vi "Main.vi"(8 "error":errorcluster) -> (0 "Error out":errorcluster)   [LabVIEW 2018, in "GUI.lvclass"]
uses:
  GUI.lvclass
  Public Controls/GlobalConfig.ctl
  Public Controls/S1Config.ctl
  Public Controls/S2Config.ctl
  Public Controls/TestInfo.ctl
  GUI.lvclass/GUI.ctl
  <vilib>/DAQmx/write.llb/DAQmx Write (Digital Bool 1Line 1Point).vi
  <vilib>/DAQmx/miscellaneous.llb/DAQmx Fill In Error Info.vi
  S1/S1.lvclass
  S2/S2.lvclass
  IO/IO.lvclass
  S3/S3.lvclass
  S4/S4.lvclass
  S5/S5.lvclass
  S6/S6.lvclass
  Serial/Serial.lvclass
panel:
  in  "Tab Control":T1(tab)
  out "S2 Valves":bool[](array[boolean])
  out "S1 Valves":bool[](array[boolean])
  out "EC_PTEST_DELTA_MAX":dbl format="%.2f psig"
  in  "S2AckAlarm":bool
  in  "S1AckAlarm":bool
  out "PRESSURE PT1":dbl(knob) scale=0.0..400.0
  out "PRESSURE PT1":dbl(knob) scale=0.0..400.0 scale format="%_3g"
  in  "ABORT1":bool
  out "ELAPSED TIME 2":dbl caption="REMAINING STATE TIME" format="%<%H:%M:%S>t"
  out "IsLidLocked 2":bool caption="IsLidLocked"
  in  "SN 2":string caption="SN"
  in  "S2Start":bool
  out "IsLidLocked":bool
  in  "S1Start":bool
  in  "SN":string
  in  "ABORT 2":bool
  out "ELAPSED TIME 1":dbl caption="REMAINING STATE TIME" format="%<%H:%M:%S>t"
  out "TEST STOPPED AT:":string
  out "S1 TEST STARTED AT:":string caption="TEST STARTED AT:"
  out "2 TEST STOPPED AT:":string caption="TEST STOPPED AT:"
  out "2 TEST STARTED AT:":string caption="TEST STARTED AT:"
  out "PRESSURE PT231":dbl(knob) scale=0.0..400.0
  out "PRESSURE PT221":dbl(knob) scale=0.0..400.0
  out "TEST RESULT 2":string caption="TEST RESULT"
  out "TEST STATE":string
  out "Pressure vs Time Plot 2":waveform(dbl)[](graph)
  out "TEST STATUS 2":string caption="TEST STATUS"
  in  "Select Test Type 2":string(combo) caption="Test Type"
  out "PRESSURE PT131":dbl(knob) scale=0.0..0.5 scale format="%_3g"
  out "PRESSURE PT121":dbl(knob) scale=0.0..400.0 scale format="%#.3g"
  out "PRESSURE PT111":dbl(knob) scale=0.0..400.0 scale format="%#.3g"
  out "TEST RESULT 1":string caption="TEST RESULT"
  out "CURRENT TEST STATE 1":string caption="TEST STATE"
  out "Pressure vs Time Plot 1":waveform(dbl)[](graph)
  out "TEST STATUS 1":string caption="TEST STATUS"
  in  "Test Type 1":string(combo) caption="Test Type"
  in  "LidLock-Extend(SV615)":bool
  in  "Z2 Vent(SV621)":bool
  in  "LidLock-Retract(SV614)":bool
  in  "Z3 Vent(SV633)":bool
  in  "Hi Pressure N2(SV632)":bool
  in  "Lo Pressure N2(SV631)":bool
  out "CPS612":bool
  out "CPS611":bool
  in  "LidLock-Extend(SV515)":bool
  in  "Z2 Vent(SV521)":bool
  in  "LidLock-Retract(SV514)":bool
  in  "Z3 Vent(SV533)":bool
  in  "Hi Pressure N2(SV532)":bool
  in  "Lo Pressure N2(SV531)":bool
  out "CPS512":bool
  out "CPS511":bool
  in  "LidLock-Extend(SV415)":bool
  in  "Z2 Vent(SV421)":bool
  in  "LidLock-Retract(SV414)":bool
  in  "Z3 Vent(SV433)":bool
  in  "Hi Pressure N2(SV432)":bool
  in  "Lo Pressure N2(SV431)":bool
  out "CPS412":bool
  out "CPS411":bool
  in  "LidLock-Extend(SV315)":bool
  in  "Z2 Vent(SV321)":bool
  in  "LidLock-Retract(SV314)":bool
  in  "Z3 Vent(SV333)":bool
  in  "Hi Pressure N2(SV332)":bool
  in  "Lo Pressure N2(SV331)":bool
  out "CPS312":bool
  out "CPS311":bool
  in  "LidLock-Extend(SV215)":bool
  in  "Z2 Vent(SV221)":bool
  in  "LidLock-Retract(SV214)":bool
  in  "Z3 Vent(SV233)":bool
  in  "LidLock-Retract(SV114)":bool
  in  "LidLock-Extend(SV115)":bool
  in  "Hi Pressure N2(SV232)":bool
  in  "Lo Pressure N2(SV231)":bool
  in  "Z3 Vent(SV131)":bool
  in  "Lo Pressure N2(SV111)":bool
  out "CPS212":bool
  out "CPS211":bool
  out "CPS112":bool
  out "CPS111":bool
  in  "Z1 Vent(SV113)":bool
  in  "Hi Pressure N2(SV112)":bool
  in  "Z2 Vent(SV121)":bool
  in  "Global":T2={"Report Folder Path"=path "", "PT1_MIN"=0.0, "PT1_MAX"=0.0, "VENT_PMAX"=0.0, "LOP_TARGET"=0.0, "LOP_RAMP"=0.0, "LOP_LEAK_MAX"=0.0, "HIP_TARGET"=0.0, "HIP_RAMP"=0.0, "HIP_MIN"=0.0, "HIP_MAX"=0.0, "BLEED_TIME"=0.0, "LOP_MAX"=0.0, "LOP_MIN"=0.0, "PT131Com"="COM5", "PT231Com"="COM6", "PT331Com"="COM7", "PT431Com"="COM8", "PT531Com"="COM9", "PT631Com"="COM10"} {"LOP_MIN" format="%#_g PSI"; "LOP_MAX" format="%#_g PSI"; "BLEED_TIME" format="%#_g Sec"; "HIP_MAX" format="%#_g PSI"; "HIP_MIN" format="%#_g PSI"; "HIP_RAMP" format="%#_g Sec"; "HIP_TARGET" format="%#_g PSI"; "LOP_LEAK_MAX" format="%#_g PSI"; "LOP_RAMP" format="%#_g Sec"; "LOP_TARGET" format="%#_g PSI"; "VENT_PMAX" format="%#_g PSI"; "PT1_MAX" format="%#_g PSI"; "PT1_MIN" format="%#_g PSI"}
  in  "S1Config":T3 {"TJHIP_STABLE_CLOSE" format="%#_g sec"; "TJHIP_STABLE_WAIT" format="%#_g sec"; "TJ_PTEST_MAX" format="%#_g in H20"; "TJHIP_TIMER" format="%#_g sec"; "TJLOP_TIMER" format="%#_g sec"; "MSHIP_TIMER" format="%#_g sec"; "S1Z3_LOP_LEAK_MAX" format="%#_g in H20"; "MSLOP_TIMER" format="%#_g sec"; "S1Z3_VENT_PMAX" format="%#_g in H20"}
  in  "Station 6":T4 {"EC_PTEST_DELTA_BASELINE" format="%#_g psi"; "EC_PTEST_SCALE_FACTOR" min=0.0 max=1.0 step=0.01; "ECZ3_POFF_STABLE" format="%#_g sec"; "EC_PSTABLE_WAIT" format="%#_g sec"; "EC_PTEST_TIMER" format="%#_g sec"; "ECLOP_TIMER" format="%#_g sec"}
  in  "Station 5":T4 {"EC_PTEST_DELTA_BASELINE" format="%#_g psi"; "EC_PTEST_SCALE_FACTOR" min=0.0 max=1.0 step=0.01; "ECZ3_POFF_STABLE" format="%#_g sec"; "EC_PSTABLE_WAIT" format="%#_g sec"; "EC_PTEST_TIMER" format="%#_g sec"; "ECLOP_TIMER" format="%#_g sec"}
  in  "Station 4":T4 {"EC_PTEST_DELTA_BASELINE" format="%#_g psi"; "EC_PTEST_SCALE_FACTOR" min=0.0 max=1.0 step=0.01; "ECZ3_POFF_STABLE" format="%#_g sec"; "EC_PSTABLE_WAIT" format="%#_g sec"; "EC_PTEST_TIMER" format="%#_g sec"; "ECLOP_TIMER" format="%#_g sec"}
  in  "Station 3":T4 {"EC_PTEST_DELTA_BASELINE" format="%#_g psi"; "EC_PTEST_SCALE_FACTOR" min=0.0 max=1.0 step=0.01; "ECZ3_POFF_STABLE" format="%#_g sec"; "EC_PSTABLE_WAIT" format="%#_g sec"; "EC_PTEST_TIMER" format="%#_g sec"; "ECLOP_TIMER" format="%#_g sec"}
  in  "Station 2":T4 {"EC_PTEST_DELTA_BASELINE" format="%#_g psi"; "EC_PTEST_SCALE_FACTOR" min=0.0 max=1.0 step=0.01; "ECZ3_POFF_STABLE" format="%#_g sec"; "EC_PSTABLE_WAIT" format="%#_g sec"; "EC_PTEST_TIMER" format="%#_g sec"; "ECLOP_TIMER" format="%#_g sec"}
  # "Version 2.0.0"
  # "This template is for the Simple State Machine design pattern.\n\nSee the block diagram for more information on how to use this template."
  # "STATION #1"
  # "STATION #2"
  # "LoP"
  # "HiP"
  # "Z1"
  # "Z2"
  # "Z3"
  # "Lid Ext"
  # "LoP"
  # "HiP"
  # "Z3"
  # "Z2"
  # "Lid Ext"
  # "STATION 1"
  # "STATION 2"
  # "STATION 4"
  # "STATION 5"
  # "STATION 6"
  # "STATION 3"
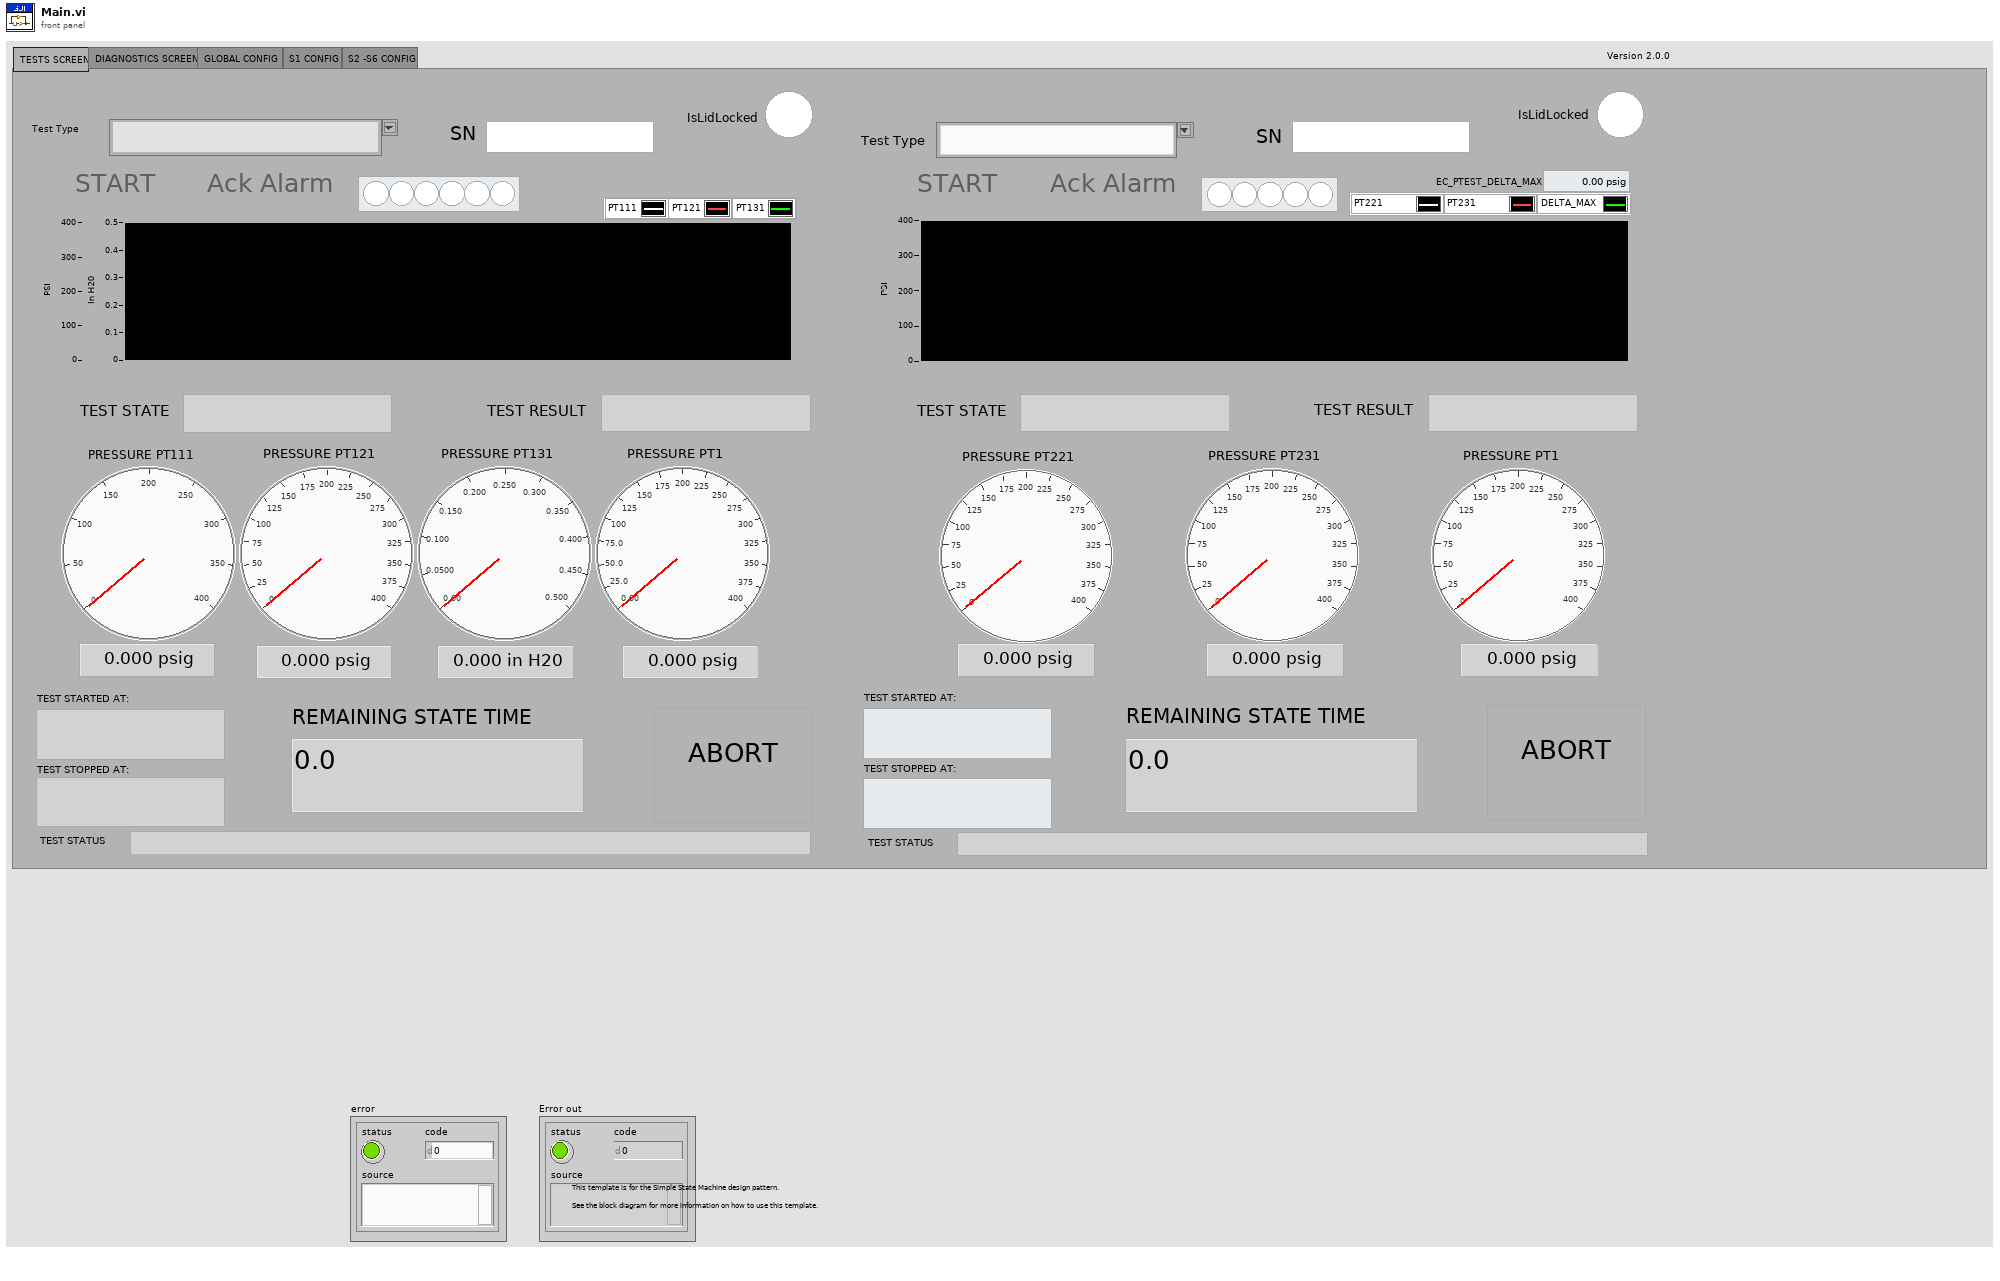
[diagram p1: front panel]
types:
  T1 = enum32{"TESTS SCREEN", "DIAGNOSTICS SCREEN", "GLOBAL CONFIG", "S1 CONFIG", "S2 -S6 CONFIG"}
  T2 = typedef "GUI.lvclass/GlobalConfig.ctl" = cluster{"Report Folder Path":path, "PT1_MIN":dbl, "PT1_MAX":dbl, "VENT_PMAX":dbl, "LOP_TARGET":dbl, "LOP_RAMP":dbl, "LOP_LEAK_MAX":dbl, "HIP_TARGET":dbl, "HIP_RAMP":dbl, "HIP_MIN":dbl, "HIP_MAX":dbl, "BLEED_TIME":dbl, "LOP_MAX":dbl, "LOP_MIN":dbl, "PT131Com":refnum<visa-resource-name>, "PT231Com":refnum<visa-resource-name>, "PT331Com":refnum<visa-resource-name>, "PT431Com":refnum<visa-resource-name>, "PT531Com":refnum<visa-resource-name>, "PT631Com":refnum<visa-resource-name>}
  T3 = typedef "GUI.lvclass/S1Config.ctl" = cluster{"S1Z3_VENT_PMAX":dbl, "MSLOP_TIMER":dbl, "S1Z3_LOP_LEAK_MAX":dbl, "MSHIP_TIMER":dbl, "TJLOP_TIMER":dbl, "TJHIP_TIMER":dbl, "TJ_PTEST_MAX":dbl, "TJHIP_STABLE_WAIT":dbl, "TJHIP_STABLE_CLOSE":dbl}
  T4 = typedef "GUI.lvclass/S2Config.ctl" = cluster{"ECLOP_TIMER":dbl, "EC_PTEST_TIMER":dbl, "EC_PSTABLE_WAIT":dbl, "ECZ3_POFF_STABLE":dbl, "EC_PTEST_SCALE_FACTOR":dbl, "EC_PTEST_DELTA_BASELINE":dbl}
  T5 = enum8{"Enabled", "Disabled", "Disabled and Grayed Out"}
  T6 = typedef "GUI.lvclass/TestInfo.ctl" = cluster{"TestType":string, "SN":string}
  T7 = typedef "GUI.lvclass/State.ctl" = enum16{"Initialize", "LoadConfig", "SaveConfig", "S1Alarm", "S2Alarm", "S1EndOfTest", "S2EndOfTest", "Monitor", "Error", "Exit"}
  T8 = cluster{"Global":T2, "S1Config":T3, "Station 2 ":T4, "Station 3":T4, "Station 4":T4, "Station 5":T4, "Station 6":T4}
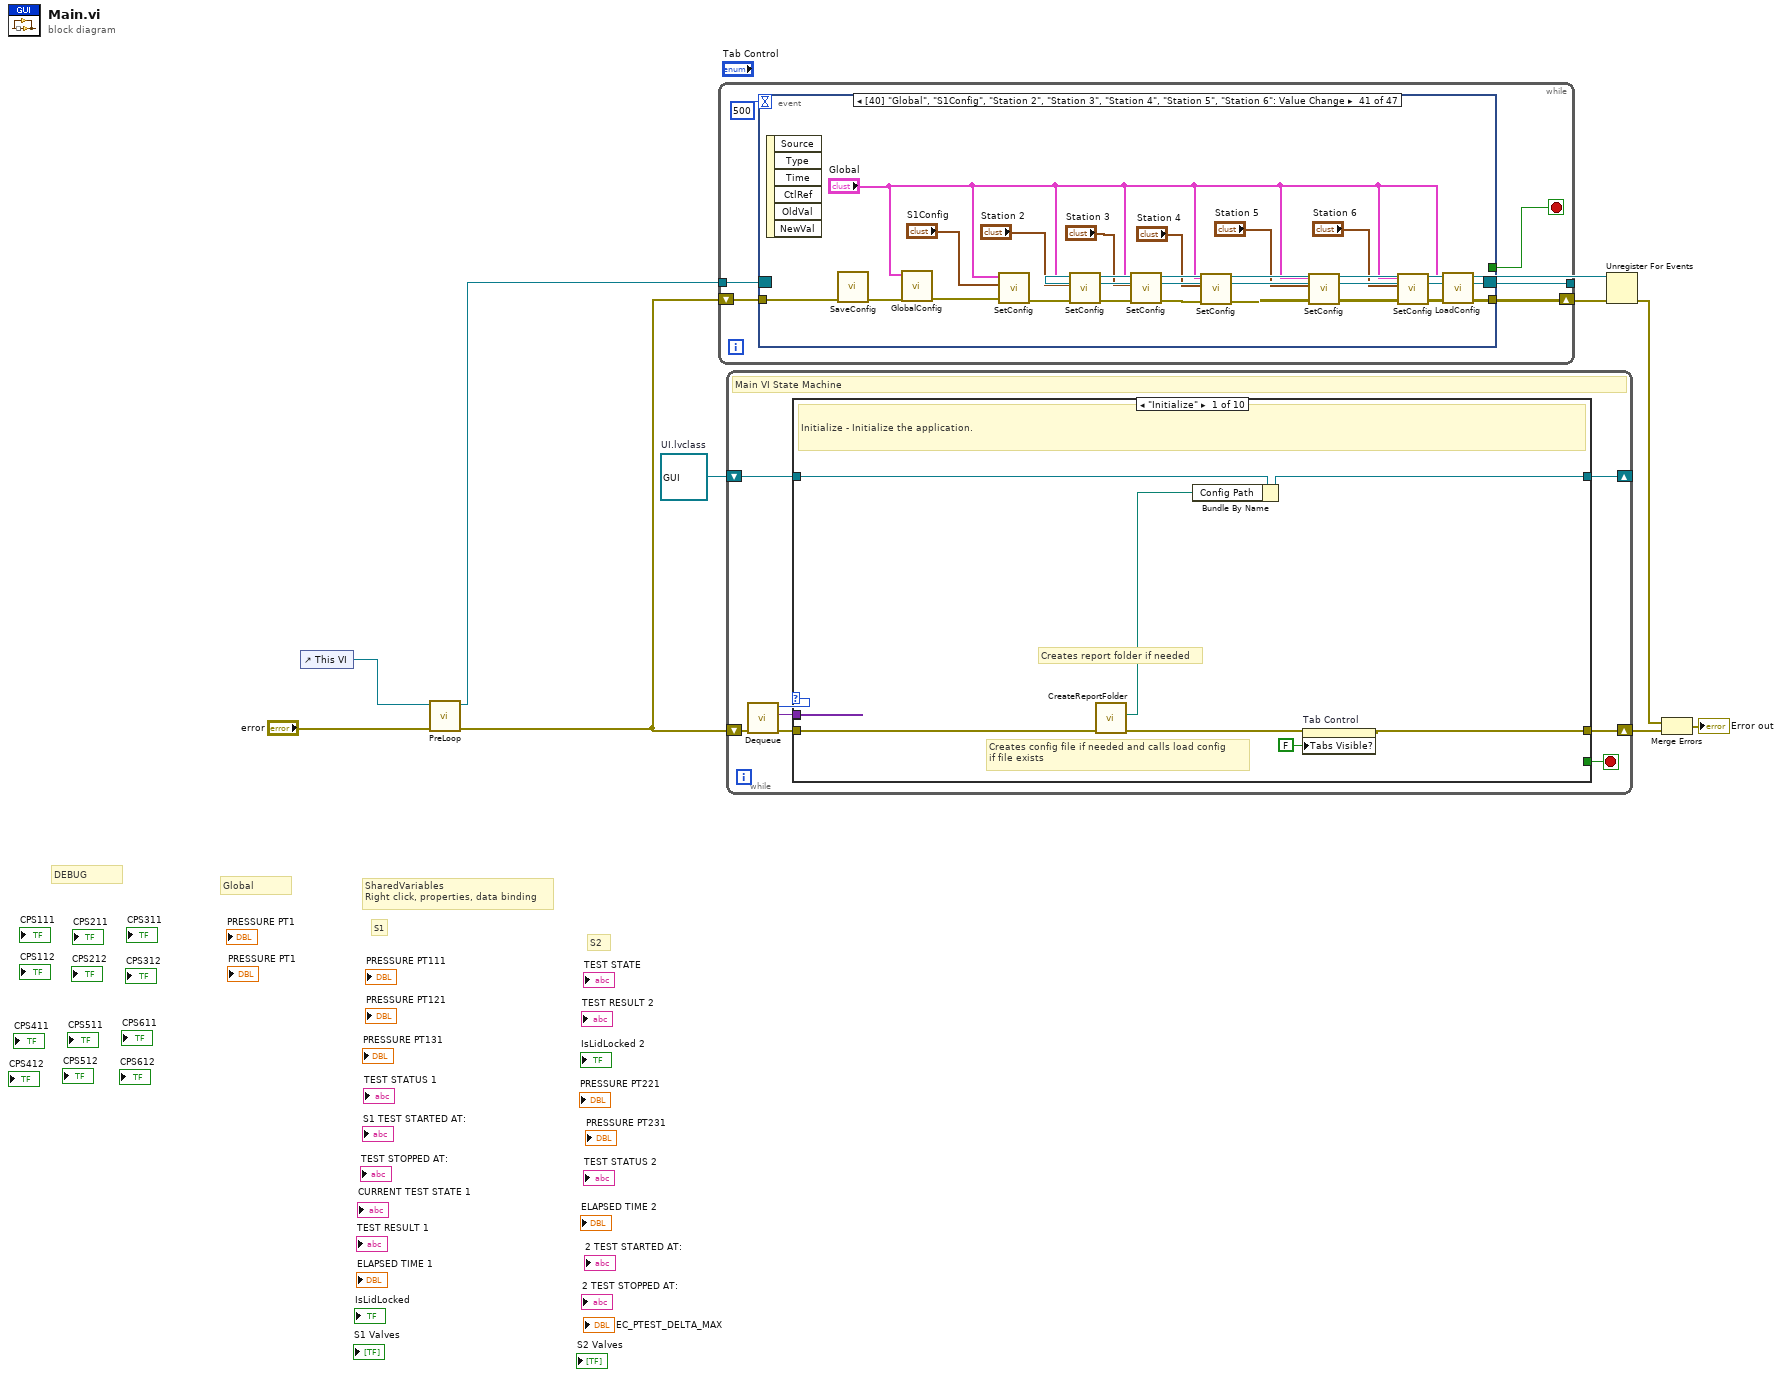
[diagram p0: block diagram]
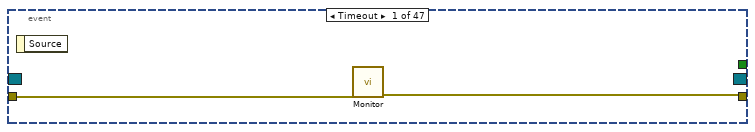
[diagram p2: hidden frame]
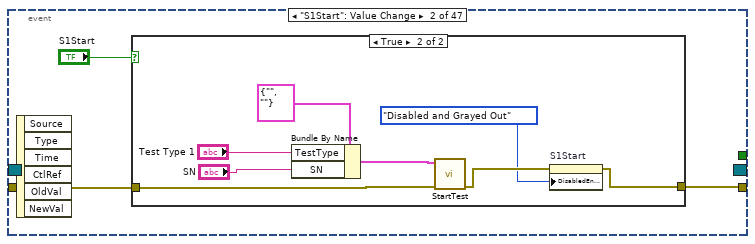
[diagram p3: hidden frame]
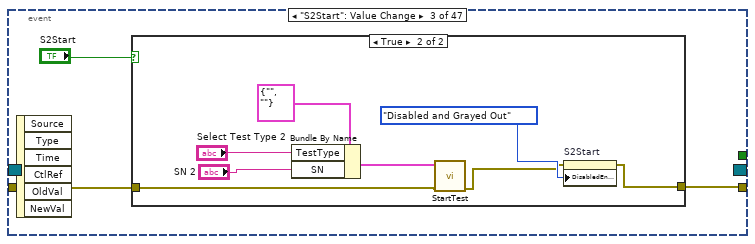
[diagram p5: hidden frame]
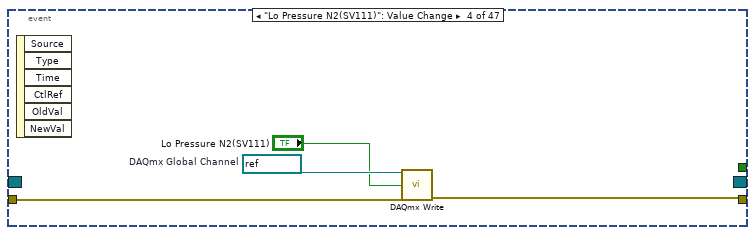
[diagram p7: hidden frame]
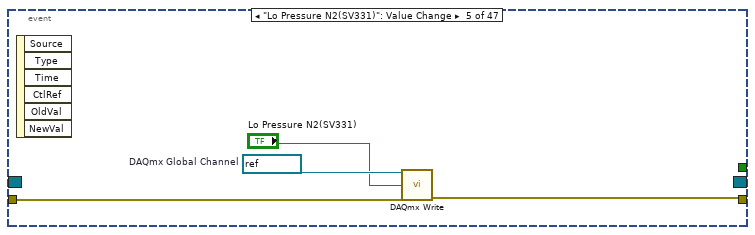
[diagram p8: hidden frame]
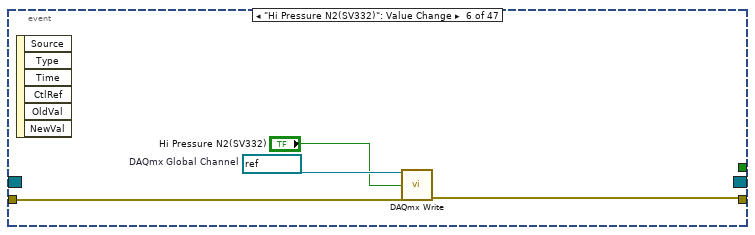
[diagram p9: hidden frame]
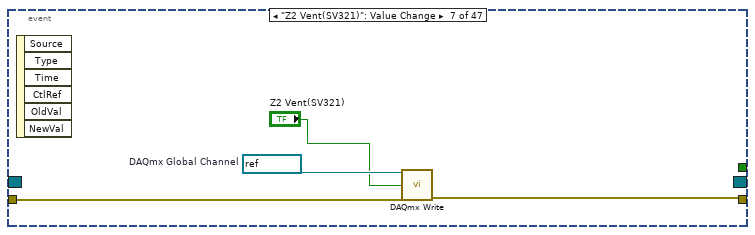
[diagram p10: hidden frame]
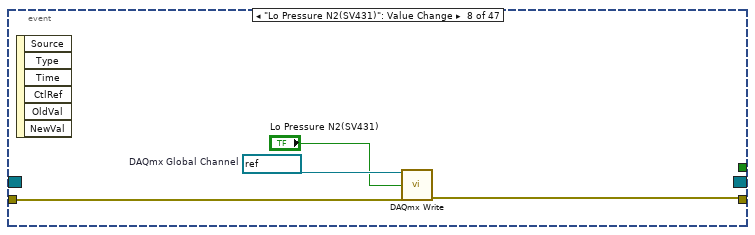
[diagram p11: hidden frame]
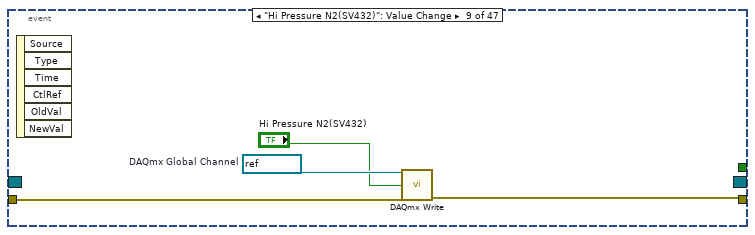
[diagram p12: hidden frame]
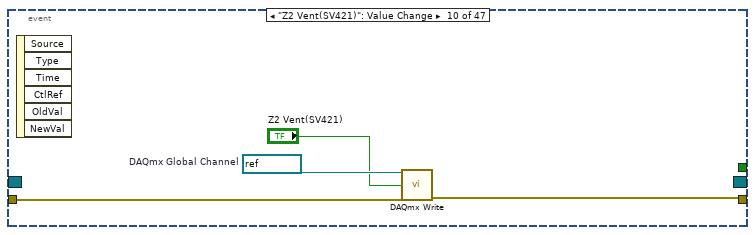
[diagram p13: hidden frame]
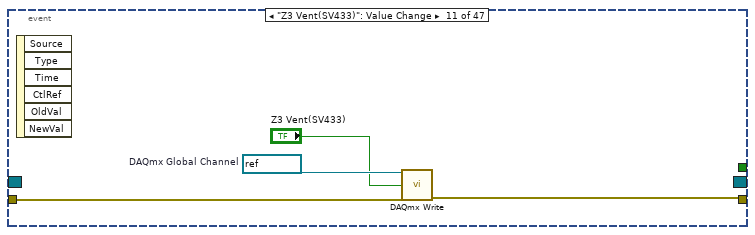
[diagram p14: hidden frame]
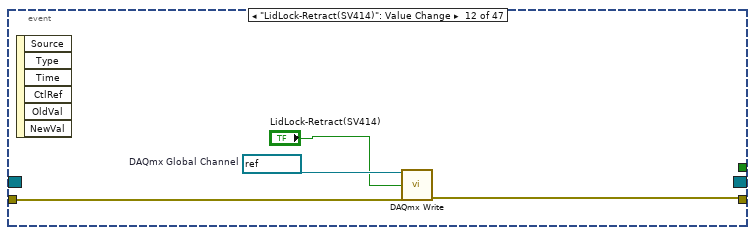
[diagram p15: hidden frame]
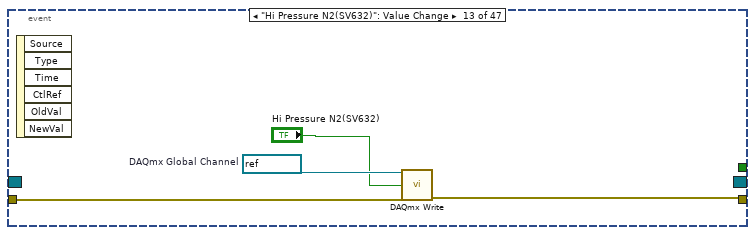
[diagram p16: hidden frame]
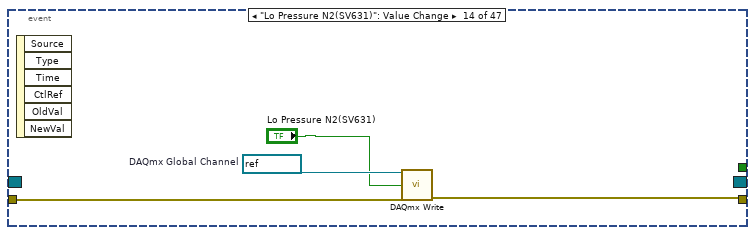
[diagram p17: hidden frame]
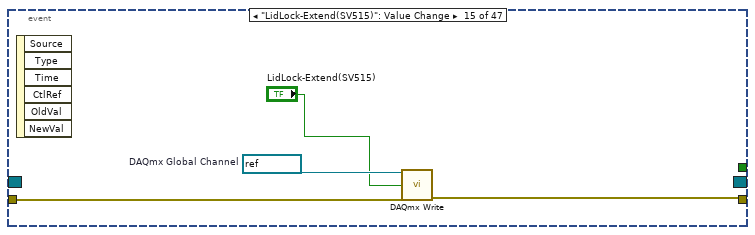
[diagram p18: hidden frame]
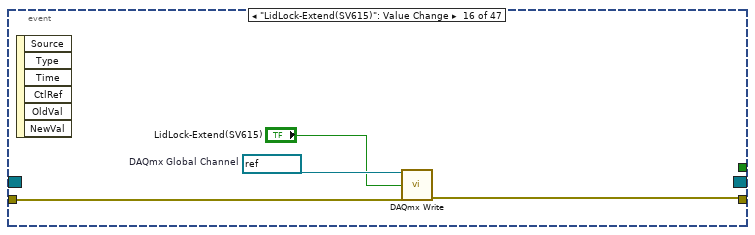
[diagram p19: hidden frame]
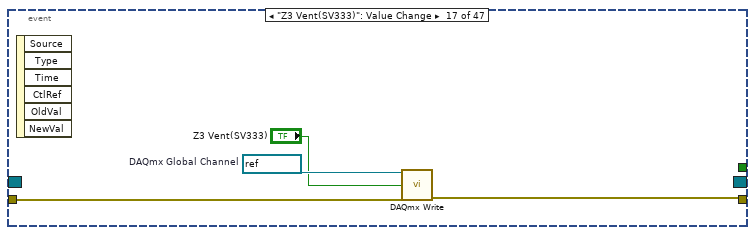
[diagram p20: hidden frame]
diagram:
  w10 = refnum<class "GUI.lvclass"> refnum  # UI.lvclass
  # "Global"
  # "S2"
  # "DEBUG"
  # "S1"
  # "SharedVariables\nRight click, properties, data binding"
  n1 = control-ref of="This VI"() -> (w4:refnum<vi>)
  n2 = call "PreLoop.vi"("error in"="error", "VI Ref"=w4) -> ("error out"=w2:errorcluster, "Event Out"=w1:refnum<event-registration>)  [unwired: 8 in]
  n3 = while {
    shift-right: [w14] -> w9
    shift-left: w2 -> [w16]
    tunnel: [w13] -> w8
    tunnel: w1 -> [w11]
    stop <- w15 stop-if-true
    n4 = event shown="[40] \"Global\", \"S1Config\", \"Station 2\", \"Station 3\", \"Station 4\", \"Station 5\", \"Station 6\": Value Change" {
      selector: w11 -> [_ _ _ _ _ _ _ _ _ _ _ _ _ _ _ _ _ _ _ _ _ _ _ _ _ _ _ _ _ _ _ _ _ _ _ _ _ _ _ _ _ _ _ _ _ _ _]
      dyn-events: [_ _ _ _ _ _ _ _ _ _ _ _ _ _ _ _ _ _ _ _ _ _ _ _ _ _ _ _ _ _ _ _ _ _ _ _ _ _ _ _ _ _ _ _ _ _ _] -> w13
      timeout: 500 -> [_ _ _ _ _ _ _ _ _ _ _ _ _ _ _ _ _ _ _ _ _ _ _ _ _ _ _ _ _ _ _ _ _ _ _ _ _ _ _ _ _ _ _ _ _ _ _]
      tunnel: w16 -> [w18 w21 w33 w45 w49 w53 w57 w61 w65 w69 w73 w77 w81 w85 w89 w93 w97 w101 w105 w109 w113 w117 w121 w125 w129 w133 w137 w141 w145 w149 w153 w157 w161 w165 w169 w173 w177 w181 w185 w189 w207 w209 w218 w224 w229 w235 w242]
      tunnel: [w17 w20 w32 w44 w48 w52 w56 w60 w64 w68 w72 w76 w80 w84 w88 w92 w96 w100 w104 w108 w112 w116 w120 w124 w128 w132 w136 w140 w144 w148 w152 w156 w160 w164 w168 w172 w176 w180 w184 w188 w191 w209 w217 w222 w228 w234 w241] -> w14
      tunnel: [_ _ _ _ _ _ _ _ _ _ _ _ _ _ _ _ _ _ _ _ _ _ _ _ _ _ _ _ _ _ _ _ _ _ _ _ _ _ _ _ _ _ _ _ _ _ TRUE] -> w15
      event Timeout {
        n5 = event-data() -> ()  [unwired: 1 in, 1 out]
        n6 = call "Monitor.vi"("error in"=w18) -> ("error out"=w17:errorcluster)  [unwired: 10 in]
      }
      event "S1Start": Value Change {
        n7 = event-data() -> ()  [unwired: 1 in, 6 out]
        n8 = case shown="True" "S1Start" {
          tunnel: w21 -> [w22 w26]
          tunnel: [w22 w23] -> w20
          frame False {
          }
          frame True {
            n9 = Bundle By Name(cluster=T6 {"TestType"="", "SN"=""}, "TestType"="Test Type 1", "SN"="SN") -> (w27:T6)
            n10 = call "StartTest.vi"("error in"=w26, "TestInfo"=w27) -> ("error out"=w25:errorcluster)  [unwired: 9 in]
            n11 = property on="S1Start" class="Bool"(error in=w25, "DisabledEnum"=T5."Disabled and Grayed Out" ("Disabled")) -> (error out=w23:errorcluster)  [unwired: 1 in, 1 out]
          }
        }
      }
      event "S2Start": Value Change {
        n12 = event-data() -> ()  [unwired: 1 in, 6 out]
        n13 = case shown="True" "S2Start" {
          tunnel: w33 -> [w34 w37]
          tunnel: [w34 w39] -> w32
          frame False {
          }
          frame True {
            n14 = Bundle By Name(cluster=T6 {"TestType"="", "SN"=""}, "TestType"="Select Test Type 2", "SN"="SN 2") -> (w38:T6)
            n15 = call "StartTest.vi"("error in"=w37, "TestInfo"=w38) -> ("error out"=w36:errorcluster)  [unwired: 9 in]
            n16 = property on="S2Start" class="Bool"(error in=w36, "DisabledEnum"=T5."Disabled and Grayed Out" ("Disabled")) -> (error out=w39:errorcluster)  [unwired: 1 in, 1 out]
          }
        }
      }
      event "Lo Pressure N2(SV111)": Value Change {
        w46 = refnum<k21> "SV111"  # DAQmx Global Channel
        n17 = event-data() -> ()  [unwired: 1 in, 6 out]
        n18 = call-poly <vilib>:"DAQmx Write.vi"("task/channels in"=w46, "data"="Lo Pressure N2(SV111)", "error in"=w45) -> ("error out"=w44:errorcluster)  [unwired: 10 in, 2 out]
      }
      event "Lo Pressure N2(SV331)": Value Change {
        w50 = refnum<k21> "SV331"  # DAQmx Global Channel
        n19 = event-data() -> ()  [unwired: 1 in, 6 out]
        n20 = call-poly <vilib>:"DAQmx Write.vi"("task/channels in"=w50, "data"="Lo Pressure N2(SV331)", "error in"=w49) -> ("error out"=w48:errorcluster)  [unwired: 10 in, 2 out]
      }
      event "Hi Pressure N2(SV332)": Value Change {
        w54 = refnum<k21> "SV332"  # DAQmx Global Channel
        n21 = event-data() -> ()  [unwired: 1 in, 6 out]
        n22 = call-poly <vilib>:"DAQmx Write.vi"("task/channels in"=w54, "data"="Hi Pressure N2(SV332)", "error in"=w53) -> ("error out"=w52:errorcluster)  [unwired: 10 in, 2 out]
      }
      event "Z2 Vent(SV321)": Value Change {
        w58 = refnum<k21> "SV321"  # DAQmx Global Channel
        n23 = event-data() -> ()  [unwired: 1 in, 6 out]
        n24 = call-poly <vilib>:"DAQmx Write.vi"("task/channels in"=w58, "data"="Z2 Vent(SV321)", "error in"=w57) -> ("error out"=w56:errorcluster)  [unwired: 10 in, 2 out]
      }
      event "Lo Pressure N2(SV431)": Value Change {
        w62 = refnum<k21> "SV431"  # DAQmx Global Channel
        n25 = event-data() -> ()  [unwired: 1 in, 6 out]
        n26 = call-poly <vilib>:"DAQmx Write.vi"("task/channels in"=w62, "data"="Lo Pressure N2(SV431)", "error in"=w61) -> ("error out"=w60:errorcluster)  [unwired: 10 in, 2 out]
      }
      event "Hi Pressure N2(SV432)": Value Change {
        w66 = refnum<k21> "SV432"  # DAQmx Global Channel
        n27 = event-data() -> ()  [unwired: 1 in, 6 out]
        n28 = call-poly <vilib>:"DAQmx Write.vi"("task/channels in"=w66, "data"="Hi Pressure N2(SV432)", "error in"=w65) -> ("error out"=w64:errorcluster)  [unwired: 10 in, 2 out]
      }
      event "Z2 Vent(SV421)": Value Change {
        w70 = refnum<k21> "SV421"  # DAQmx Global Channel
        n29 = event-data() -> ()  [unwired: 1 in, 6 out]
        n30 = call-poly <vilib>:"DAQmx Write.vi"("task/channels in"=w70, "data"="Z2 Vent(SV421)", "error in"=w69) -> ("error out"=w68:errorcluster)  [unwired: 10 in, 2 out]
      }
      event "Z3 Vent(SV433)": Value Change {
        w74 = refnum<k21> "SV433"  # DAQmx Global Channel
        n31 = event-data() -> ()  [unwired: 1 in, 6 out]
        n32 = call-poly <vilib>:"DAQmx Write.vi"("task/channels in"=w74, "data"="Z3 Vent(SV433)", "error in"=w73) -> ("error out"=w72:errorcluster)  [unwired: 10 in, 2 out]
      }
      event "LidLock-Retract(SV414)": Value Change {
        w78 = refnum<k21> "SV414"  # DAQmx Global Channel
        n33 = event-data() -> ()  [unwired: 1 in, 6 out]
        n34 = call-poly <vilib>:"DAQmx Write.vi"("task/channels in"=w78, "data"="LidLock-Retract(SV414)", "error in"=w77) -> ("error out"=w76:errorcluster)  [unwired: 10 in, 2 out]
      }
      event "Hi Pressure N2(SV632)": Value Change {
        w82 = refnum<k21> "SV632"  # DAQmx Global Channel
        n35 = event-data() -> ()  [unwired: 1 in, 6 out]
        n36 = call-poly <vilib>:"DAQmx Write.vi"("task/channels in"=w82, "data"="Hi Pressure N2(SV632)", "error in"=w81) -> ("error out"=w80:errorcluster)  [unwired: 10 in, 2 out]
      }
      event "Lo Pressure N2(SV631)": Value Change {
        w86 = refnum<k21> "SV631"  # DAQmx Global Channel
        n37 = event-data() -> ()  [unwired: 1 in, 6 out]
        n38 = call-poly <vilib>:"DAQmx Write.vi"("task/channels in"=w86, "data"="Lo Pressure N2(SV631)", "error in"=w85) -> ("error out"=w84:errorcluster)  [unwired: 10 in, 2 out]
      }
      event "LidLock-Extend(SV515)": Value Change {
        w90 = refnum<k21> "SV515"  # DAQmx Global Channel
        n39 = event-data() -> ()  [unwired: 1 in, 6 out]
        n40 = call-poly <vilib>:"DAQmx Write.vi"("task/channels in"=w90, "data"="LidLock-Extend(SV515)", "error in"=w89) -> ("error out"=w88:errorcluster)  [unwired: 10 in, 2 out]
      }
      event "LidLock-Extend(SV615)": Value Change {
        w94 = refnum<k21> "SV615"  # DAQmx Global Channel
        n41 = event-data() -> ()  [unwired: 1 in, 6 out]
        n42 = call-poly <vilib>:"DAQmx Write.vi"("task/channels in"=w94, "data"="LidLock-Extend(SV615)", "error in"=w93) -> ("error out"=w92:errorcluster)  [unwired: 10 in, 2 out]
      }
      event "Z3 Vent(SV333)": Value Change {
        w98 = refnum<k21> "SV333"  # DAQmx Global Channel
        n43 = event-data() -> ()  [unwired: 1 in, 6 out]
        n44 = call-poly <vilib>:"DAQmx Write.vi"("task/channels in"=w98, "data"="Z3 Vent(SV333)", "error in"=w97) -> ("error out"=w96:errorcluster)  [unwired: 10 in, 2 out]
      }
      event "LidLock-Retract(SV314)": Value Change {
        w102 = refnum<k21> "SV314"  # DAQmx Global Channel
        n45 = event-data() -> ()  [unwired: 1 in, 6 out]
        n46 = call-poly <vilib>:"DAQmx Write.vi"("task/channels in"=w102, "data"="LidLock-Retract(SV314)", "error in"=w101) -> ("error out"=w100:errorcluster)  [unwired: 10 in, 2 out]
      }
      event "LidLock-Extend(SV415)": Value Change {
        w106 = refnum<k21> "SV415"  # DAQmx Global Channel
        n47 = event-data() -> ()  [unwired: 1 in, 6 out]
        n48 = call-poly <vilib>:"DAQmx Write.vi"("task/channels in"=w106, "data"="LidLock-Extend(SV415)", "error in"=w105) -> ("error out"=w104:errorcluster)  [unwired: 10 in, 2 out]
      }
      event "Z3 Vent(SV633)": Value Change {
        w110 = refnum<k21> "SV633"  # DAQmx Global Channel
        n49 = event-data() -> ()  [unwired: 1 in, 6 out]
        n50 = call-poly <vilib>:"DAQmx Write.vi"("task/channels in"=w110, "data"="Z3 Vent(SV633)", "error in"=w109) -> ("error out"=w108:errorcluster)  [unwired: 10 in, 2 out]
      }
      event "Z2 Vent(SV521)": Value Change {
        w114 = refnum<k21> "SV521"  # DAQmx Global Channel
        n51 = event-data() -> ()  [unwired: 1 in, 6 out]
        n52 = call-poly <vilib>:"DAQmx Write.vi"("task/channels in"=w114, "data"="Z2 Vent(SV521)", "error in"=w113) -> ("error out"=w112:errorcluster)  [unwired: 10 in, 2 out]
      }
      event "Lo Pressure N2(SV531)": Value Change {
        w118 = refnum<k21> "SV531"  # DAQmx Global Channel
        n53 = event-data() -> ()  [unwired: 1 in, 6 out]
        n54 = call-poly <vilib>:"DAQmx Write.vi"("task/channels in"=w118, "data"="Lo Pressure N2(SV531)", "error in"=w117) -> ("error out"=w116:errorcluster)  [unwired: 10 in, 2 out]
      }
      event "Hi Pressure N2(SV532)": Value Change {
        w122 = refnum<k21> "SV532"  # DAQmx Global Channel
        n55 = event-data() -> ()  [unwired: 1 in, 6 out]
        n56 = call-poly <vilib>:"DAQmx Write.vi"("task/channels in"=w122, "data"="Hi Pressure N2(SV532)", "error in"=w121) -> ("error out"=w120:errorcluster)  [unwired: 10 in, 2 out]
      }
      event "LidLock-Retract(SV514)": Value Change {
        w126 = refnum<k21> "SV514"  # DAQmx Global Channel
        n57 = event-data() -> ()  [unwired: 1 in, 6 out]
        n58 = call-poly <vilib>:"DAQmx Write.vi"("task/channels in"=w126, "data"="LidLock-Retract(SV514)", "error in"=w125) -> ("error out"=w124:errorcluster)  [unwired: 10 in, 2 out]
      }
      event "LidLock-Extend(SV315)": Value Change {
        w130 = refnum<k21> "SV315"  # DAQmx Global Channel
        n59 = event-data() -> ()  [unwired: 1 in, 6 out]
        n60 = call-poly <vilib>:"DAQmx Write.vi"("task/channels in"=w130, "data"="LidLock-Extend(SV315)", "error in"=w129) -> ("error out"=w128:errorcluster)  [unwired: 10 in, 2 out]
      }
      event "Z3 Vent(SV533)": Value Change {
        w134 = refnum<k21> "SV533"  # DAQmx Global Channel
        n61 = event-data() -> ()  [unwired: 1 in, 6 out]
        n62 = call-poly <vilib>:"DAQmx Write.vi"("task/channels in"=w134, "data"="Z3 Vent(SV533)", "error in"=w133) -> ("error out"=w132:errorcluster)  [unwired: 10 in, 2 out]
      }
      event "LidLock-Retract(SV614)": Value Change {
        w138 = refnum<k21> "SV614"  # DAQmx Global Channel
        n63 = event-data() -> ()  [unwired: 1 in, 6 out]
        n64 = call-poly <vilib>:"DAQmx Write.vi"("task/channels in"=w138, "data"="LidLock-Retract(SV614)", "error in"=w137) -> ("error out"=w136:errorcluster)  [unwired: 10 in, 2 out]
      }
      event "Z2 Vent(SV621)": Value Change {
        w142 = refnum<k21> "SV621"  # DAQmx Global Channel
        n65 = event-data() -> ()  [unwired: 1 in, 6 out]
        n66 = call-poly <vilib>:"DAQmx Write.vi"("task/channels in"=w142, "data"="Z2 Vent(SV621)", "error in"=w141) -> ("error out"=w140:errorcluster)  [unwired: 10 in, 2 out]
      }
      event "Hi Pressure N2(SV112)": Value Change {
        w146 = refnum<k21> "SV112"  # DAQmx Global Channel
        n67 = event-data() -> ()  [unwired: 1 in, 6 out]
        n68 = call-poly <vilib>:"DAQmx Write.vi"("task/channels in"=w146, "data"="Hi Pressure N2(SV112)", "error in"=w145) -> ("error out"=w144:errorcluster)  [unwired: 10 in, 2 out]
      }
      event "Z1 Vent(SV113)": Value Change {
        w150 = refnum<k21> "SV113"  # DAQmx Global Channel
        n69 = event-data() -> ()  [unwired: 1 in, 6 out]
        n70 = call-poly <vilib>:"DAQmx Write.vi"("task/channels in"=w150, "data"="Z1 Vent(SV113)", "error in"=w149) -> ("error out"=w148:errorcluster)  [unwired: 10 in, 2 out]
      }
      event "Z2 Vent(SV121)": Value Change {
        w154 = refnum<k21> "SV121"  # DAQmx Global Channel
        n71 = event-data() -> ()  [unwired: 1 in, 6 out]
        n72 = call-poly <vilib>:"DAQmx Write.vi"("task/channels in"=w154, "data"="Z2 Vent(SV121)", "error in"=w153) -> ("error out"=w152:errorcluster)  [unwired: 10 in, 2 out]
      }
      event "Z3 Vent(SV131)": Value Change {
        w158 = refnum<k21> "SV131"  # DAQmx Global Channel
        n73 = event-data() -> ()  [unwired: 1 in, 6 out]
        n74 = call-poly <vilib>:"DAQmx Write.vi"("task/channels in"=w158, "data"="Z3 Vent(SV131)", "error in"=w157) -> ("error out"=w156:errorcluster)  [unwired: 10 in, 2 out]
      }
      event "LidLock-Retract(SV114)": Value Change {
        w162 = refnum<k21> "SV114"  # DAQmx Global Channel
        n75 = event-data() -> ()  [unwired: 1 in, 6 out]
        n76 = call-poly <vilib>:"DAQmx Write.vi"("task/channels in"=w162, "data"="LidLock-Retract(SV114)", "error in"=w161) -> ("error out"=w160:errorcluster)  [unwired: 10 in, 2 out]
      }
      event "LidLock-Extend(SV115)": Value Change {
        w166 = refnum<k21> "SV115"  # DAQmx Global Channel
        n77 = event-data() -> ()  [unwired: 1 in, 6 out]
        n78 = call-poly <vilib>:"DAQmx Write.vi"("task/channels in"=w166, "data"="LidLock-Extend(SV115)", "error in"=w165) -> ("error out"=w164:errorcluster)  [unwired: 10 in, 2 out]
      }
      event "Lo Pressure N2(SV231)": Value Change {
        w170 = refnum<k21> "SV231"  # DAQmx Global Channel
        n79 = event-data() -> ()  [unwired: 1 in, 6 out]
        n80 = call-poly <vilib>:"DAQmx Write.vi"("task/channels in"=w170, "data"="Lo Pressure N2(SV231)", "error in"=w169) -> ("error out"=w168:errorcluster)  [unwired: 10 in, 2 out]
      }
      event "Hi Pressure N2(SV232)": Value Change {
        w174 = refnum<k21> "SV232"  # DAQmx Global Channel
        n81 = event-data() -> ()  [unwired: 1 in, 6 out]
        n82 = call-poly <vilib>:"DAQmx Write.vi"("task/channels in"=w174, "data"="Hi Pressure N2(SV232)", "error in"=w173) -> ("error out"=w172:errorcluster)  [unwired: 10 in, 2 out]
      }
      event "Z3 Vent(SV233)": Value Change {
        w178 = refnum<k21> "SV233"  # DAQmx Global Channel
        n83 = event-data() -> ()  [unwired: 1 in, 6 out]
        n84 = call-poly <vilib>:"DAQmx Write.vi"("task/channels in"=w178, "data"="Z3 Vent(SV233)", "error in"=w177) -> ("error out"=w176:errorcluster)  [unwired: 10 in, 2 out]
      }
      event "Z2 Vent(SV221)": Value Change {
        w182 = refnum<k21> "SV221"  # DAQmx Global Channel
        n85 = event-data() -> ()  [unwired: 1 in, 6 out]
        n86 = call-poly <vilib>:"DAQmx Write.vi"("task/channels in"=w182, "data"="Z2 Vent(SV221)", "error in"=w181) -> ("error out"=w180:errorcluster)  [unwired: 10 in, 2 out]
      }
      event "LidLock-Retract(SV214)": Value Change {
        w186 = refnum<k21> "SV214"  # DAQmx Global Channel
        n87 = event-data() -> ()  [unwired: 1 in, 6 out]
        n88 = call-poly <vilib>:"DAQmx Write.vi"("task/channels in"=w186, "data"="LidLock-Retract(SV214)", "error in"=w185) -> ("error out"=w184:errorcluster)  [unwired: 10 in, 2 out]
      }
      event "LidLock-Extend(SV215)": Value Change {
        w190 = refnum<k21> "SV215"  # DAQmx Global Channel
        n89 = event-data() -> ()  [unwired: 1 in, 6 out]
        n90 = call-poly <vilib>:"DAQmx Write.vi"("task/channels in"=w190, "data"="LidLock-Extend(SV215)", "error in"=w189) -> ("error out"=w188:errorcluster)  [unwired: 10 in, 2 out]
      }
      event Value Change {
        n91 = event-data() -> ()  [unwired: 1 in, 6 out]
        n92 = call "SaveConfig.vi"("error in"=w207) -> ("error out"=w203:errorcluster)  [unwired: 10 in]
        n93 = call "GlobalConfig.vi"("error in"=w203, "Global"="Global") -> ("error out"=w202:errorcluster)  [unwired: 9 in]
        n94 = call "SetConfig.vi"("error in"=w202, "S1Config"="S1Config", "Global"="Global") -> ("error out"=w206:errorcluster)  [unwired: 8 in]
        n95 = call "SetConfig.vi"("error in"=w206, "S2Config"="Station 2", "Global"="Global") -> ("error out"=w201:errorcluster)  [unwired: 8 in]
        n96 = call "SetConfig.vi"("error in"=w201, "S2Config"="Station 3", "Global"="Global") -> ("error out"=w200:errorcluster)  [unwired: 8 in]
        n97 = call "SetConfig.vi"("error in"=w200, "S2Config"="Station 4", "Global"="Global") -> ("error out"=w199:errorcluster)  [unwired: 8 in]
        n98 = call "SetConfig.vi"("error in"=w199, "S2Config"="Station 5", "Global"="Global") -> ("error out"=w198:errorcluster)  [unwired: 8 in]
        n99 = call "SetConfig.vi"("error in"=w198, "S2Config"="Station 6", "Global"="Global") -> ("error out"=w193:errorcluster)  [unwired: 8 in]
        n100 = call "LoadConfig.vi"("error in"=w193, "Global"="Global") -> ("error out"=w191:errorcluster)  [unwired: 9 in]
      }
      event Key Down {
        n101 = event-data() -> ("Char"=w215:i16, "PlatMods.Ctrl"=w208:bool)  [unwired: 1 in]
        n102 = Equal?(x=i16 101, y=w215) -> (x = y?=w213:bool)
        n103 = And(x=w213, y=w208) -> (x .and. y?=w212:bool)
        n104 = feedback #1() -> (w211:bool)  [unwired: 1 in]
        n105 = Not Equal?(x=w211, y=w212) -> (x != y?=w210:bool)
        n106 = feedback-in #1(w210) -> ()
        n107 = property on="Tab Control" class="TabCtl (strict)"("Tabs Visible?"=w210) -> ()  [unwired: 2 in, 2 out]
      }
      event "ABORT1": Value Change {
        n108 = event-data() -> ()  [unwired: 1 in, 1 out]
        n109 = case shown="True" "ABORT1" {
          tunnel: w218 -> [w219 w221]
          tunnel: [w219 w220] -> w217
          frame False {
          }
          frame True {
            n110 = call "Abort.vi"("error in"=w221) -> ("error out"=w220:errorcluster)  [unwired: 10 in]
          }
        }
      }
      event "ABORT 2": Value Change {
        n111 = event-data() -> ()  [unwired: 1 in, 1 out]
        n112 = case shown="True" "ABORT 2" {
          tunnel: w224 -> [w225 w227]
          tunnel: [w225 w226] -> w222
          frame False {
          }
          frame True {
            n113 = call "Abort.vi"("error in"=w227) -> ("error out"=w226:errorcluster)  [unwired: 10 in]
          }
        }
      }
      event "S1AckAlarm": Value Change {
        n114 = event-data() -> ()  [unwired: 1 in, 6 out]
        n115 = case shown="True" "S1AckAlarm" {
          tunnel: w229 -> [w231 w233]
          tunnel: [w231 w232] -> w228
          frame False {
          }
          frame True {
            n116 = call "AckAlarm.vi"("error in"=w233) -> ("error out"=w232:errorcluster)  [unwired: 10 in]
          }
        }
      }
      event "S2AckAlarm": Value Change {
        n117 = event-data() -> ()  [unwired: 1 in, 6 out]
        n118 = case shown="True" "S2AckAlarm" {
          tunnel: w235 -> [w237 w239]
          tunnel: [w237 w238] -> w234
          frame False {
          }
          frame True {
            n119 = call "AckAlarm.vi"("error in"=w239) -> ("error out"=w238:errorcluster)  [unwired: 10 in]
          }
        }
      }
      event Panel Close {
        n120 = event-data() -> ()  [unwired: 1 in, 1 out]
        n121 = call "Exit.vi"("error in"=w242) -> ("error out"=w241:errorcluster)  [unwired: 10 in]
      }
    }
  }
  n122 = while {
    shift-right: [w250] -> w7
    shift-left: w2 -> [w246]
    shift-right: [w247] -> _
    shift-left: w10 -> [w248]
    stop <- w249 stop-if-true
    # "Main VI State Machine"
    n123 = call "Dequeue.vi"("error in"=w246) -> ("error out"=w245:errorcluster, "Data"=w243:variant, "State"=w244:T7)  [unwired: 8 in]
    n124 = case shown="\"Initialize\"" w244 {
      tunnel: [_ _ _ _ _ _ _ _ w343 _] -> w249
      tunnel: w245 -> [w252 w285 w297 w309 w313 w319 w326 w335 w337 w349]
      tunnel: [w251 w275 w296 w305 w313 w314 w326 w330 w338 w345] -> w250
      tunnel: w248 -> [w257 w287 w300 w310 w312 w323 w325 w336 w342 w352]
      tunnel: [w255 w287 w300 w310 w312 w323 w325 w336 w342 w352] -> w247
      tunnel: w243 -> [_ _ _ w308 _ w318 _ _ _ w348]
      tunnel: w243 -> [_ _ _ _ _ _ _ _ _ _]
      frame "Initialize" {
        # "Creates config file if needed and calls load config\nif file exists"
        # "Creates report folder if needed"
        # "Initialize - Initialize the application."
        n125 = call "CreateReportFolder.vi"("error in (no error)"=w252) -> ("error out"=w254:errorcluster, "ConfigPath"=w253:path)  [unwired: 9 in]
        n126 = Bundle By Name(cluster=w257, "Config Path"=w253) -> (w255:refnum<class "GUI.lvclass">)
        n127 = property on="Tab Control" class="TabCtl (strict)"(error in=w254, "Tabs Visible?"=FALSE) -> (error out=w251:errorcluster)  [unwired: 1 in, 1 out]
      }
      frame "LoadConfig" {
        # "Loads the config from file"
        n128 = Unbundle By Name(w287) -> ("Config Path"=w286:path)
        n129 = Read from Text File(file (use dialog)=w286, error in=w285) -> (text=w284:string, error out=w283:errorcluster)  [unwired: 2 in, 2 out]
        n130 = local read "Station 2"() -> (w274:T4)
        n131 = local read "S1Config"() -> (w281:T3)
        n132 = local read "Station 3"() -> (w273:T4)
        n133 = local read "Station 4"() -> (w272:T4)
        n134 = local read "Station 5"() -> (w271:T4)
        n135 = local read "Station 6"() -> (w270:T4)
        n136 = local read "Global"() -> (w282:T2)
        n137 = Bundle("Global"=w282, "S1Config"=w281, "Station 2"=w274, "Station 3"=w273, "Station 4"=w272, "Station 5"=w271, "Station 6"=w270) -> (w280:T8)  [unwired: 1 in]
        n138 = Unflatten From XML(xml string=w284, type=w280, error in (no error)=w283) -> (value=w279:T8, error out=w260:errorcluster)
        n139 = Unbundle(w279) -> ("Global"=w259:T2, "S1Config"=w278:T3, "Station 2"=w276:T4, "Station 3"=w268:T4, "Station 4"=w267:T4, "Station 5"=w265:T4, "Station 6"=w261:T4)
        n140 = call "LoadConfig.vi"("error in"=w260, "Global"=w259) -> ()  [unwired: 9 in, 1 out]
        n141 = call <vilib>:"Clear Errors.vi"() -> ("error out"=w258:errorcluster)  [unwired: 6 in, 1 out]
        n142 = call "SetConfig.vi"("error in"=w258, "S1Config"=w278, "Global"=w259) -> ("error out"=w277:errorcluster)  [unwired: 8 in]
        n143 = property on="Global" class="Clust (strict)"(error in=w258, "Val(Sgnl)"=w259) -> ()  [unwired: 1 in, 2 out]
        n144 = call "SetConfig.vi"("error in"=w277, "S2Config"=w276, "Global"=w259) -> ("error out"=w269:errorcluster)  [unwired: 8 in]
        n145 = call "SetConfig.vi"("error in"=w269, "S2Config"=w268, "Global"=w259) -> ("error out"=w266:errorcluster)  [unwired: 8 in]
        n146 = call "SetConfig.vi"("error in"=w266, "S2Config"=w267, "Global"=w259) -> ("error out"=w264:errorcluster)  [unwired: 8 in]
        n147 = call "SetConfig.vi"("error in"=w264, "S2Config"=w265, "Global"=w259) -> ("error out"=w263:errorcluster)  [unwired: 8 in]
        n148 = call "SetConfig.vi"("error in"=w263, "S2Config"=w261, "Global"=w259) -> ("error out"=w262:errorcluster)  [unwired: 8 in]
        n149 = local write "Station 5"(w265) -> ()
        n150 = local write "Station 6"(w261) -> ()
        n151 = local write "S1Config"(w278) -> ()
        n152 = local write "Station 2"(w276) -> ()
        n153 = local write "Station 3"(w268) -> ()
        n154 = local write "Station 4"(w267) -> ()
        n155 = local write "Global"(w259) -> ()
        n156 = call "GlobalConfig.vi"("error in"=w262, "Global"=w259) -> ("error out"=w275:errorcluster)  [unwired: 9 in]
      }
      frame "SaveConfig" {
        # "Flatten to XML and save to file"
        n157 = local read "Station 2"() -> (w293:T4)
        n158 = local read "S1Config"() -> (w294:T3)
        n159 = local read "Station 3"() -> (w292:T4)
        n160 = local read "Station 4"() -> (w291:T4)
        n161 = local read "Station 5"() -> (w290:T4)
        n162 = local read "Station 6"() -> (w289:T4)
        n163 = local read "Global"() -> (w295:T2)
        n164 = Bundle("Global"=w295, "S1Config"=w294, "Station 2"=w293, "Station 3"=w292, "Station 4"=w291, "Station 5"=w290, "Station 6"=w289) -> (w288:T8)  [unwired: 1 in]
        n165 = Unbundle By Name(w300) -> ("Config Path"=w299:path)
        n166 = Flatten To XML(anything=w288) -> (xml string=w298:string)
        n167 = Write to Text File(file (use dialog)=w299, text=w298, error in=w297) -> (error out=w296:errorcluster)  [unwired: 1 in, 2 out]
      }
      frame "S1Alarm" {
        n168 = Variant To Data(error in=w309, type=FALSE, Variant=w308) -> (data=w304:bool, error out=w306:errorcluster)
        n169 = Select(t=T5."Disabled and Grayed Out" ("Disabled"), s=w304, f=T5."Enabled" ("Disabled")) -> (s? t:f=w301:T5)
        n170 = property on="S1AckAlarm" class="Bool"(error in=w306, "DisabledEnum"=w301, "Blinking"=w304) -> (error out=w305:errorcluster)  [unwired: 1 in, 1 out]
      }
      frame "S1EndOfTest" {
        # "Clear SN for next Test"
        n171 = local write "SN"("" ("SN")) -> ()
      }
      frame "S2Alarm" {
        n172 = Variant To Data(error in=w319, type=FALSE, Variant=w318) -> (data=w315:bool, error out=w317:errorcluster)
        n173 = Select(t=T5."Disabled and Grayed Out" ("Disabled"), s=w315, f=T5."Enabled" ("Disabled")) -> (s? t:f=w316:T5)
        n174 = property on="S2AckAlarm" class="Bool"(error in=w317, "DisabledEnum"=w316, "Blinking"=w315) -> (error out=w314:errorcluster)  [unwired: 1 in, 1 out]
      }
      frame "S2EndOfTest" {
        # "Clear SN for next Test"
        n175 = local write "SN 2"("") -> ()
      }
      frame "Monitor" {
        # "Only enable the start button if Station is in the Idle mode."
        n176 = call "DisableEnableStart.vi"() -> ("S2AckVisable"=w328:bool, "S1AckVisable"=w327:bool, "Station2"=w332:T5, "Station1"=w334:T5)  [unwired: 8 in]
        n177 = property on="S1Start" class="Bool"(error in=w335, "DisabledEnum"=w334) -> (error out=w331:errorcluster)  [unwired: 1 in, 1 out]
        n178 = property on="S2Start" class="Bool"(error in=w331, "DisabledEnum"=w332) -> (error out=w330:errorcluster)  [unwired: 1 in, 1 out]
        n179 = property on="S2AckAlarm" class="Bool"("Visible"=w328) -> ()  [unwired: 2 in, 2 out]
        n180 = property on="S1AckAlarm" class="Bool"("Visible"=w327) -> ()  [unwired: 2 in, 2 out]
        n181 = call "BuildGraph.vi"() -> ("S2"=→"Pressure vs Time Plot 2":waveform(dbl)[], "S1"=→"Pressure vs Time Plot 1":waveform(dbl)[])  [unwired: 10 in]
      }
      frame "Exit" {
        w343 = TRUE  # Stop Loop
        # "Write windows location to disc"
        # "Exit - Exit the application.\nSave / Close any files"
        n182 = call "Create Get Destroy.vi"("error In"=w337) -> ("Error Out"=w339:errorcluster, "Ref"=w341:refnum<user-event>)  [unwired: 9 in]
        n183 = Generate User Event(user event=w341, event data cluster=FALSE ("event data"), error in=w339) -> (error out=w338:errorcluster)  [unwired: 1 in, 1 out]
      }
      frame "Error" {
        n184 = Variant To Data(error in=w349, type=errorcluster {"status"=FALSE, "code"=0, "source"=""} ("error out"), Variant=w348) -> (data=w350:errorcluster, error out=w346:errorcluster)
        n185 = Unbundle By Name(w350) -> ("code"=w344:i32, "source"=w347:string)
        n186 = case shown="Default" w344 {
          tunnel: w347 -> [_ w355]
          tunnel: w346 -> [w353 w357]
          tunnel: [w353 w357] -> w345
          frame 1 {
            # "Error talking to other modules. \n\nIgnore. If testing by itself."
          }
          frame Default {
            n187 = Concatenate Strings("Error on GUI" ("message"), w355) -> (w354:string)
            n188 = One Button Dialog(message=w354) -> ()  [unwired: 1 in, 1 out]
          }
        }
      }
    }
  }
  n189 = Unregister For Events(event registration refnum=w8, error in=w9) -> (error out=w6:errorcluster)
  n190 = Merge Errors(w6, w7) -> (→"Error out":errorcluster)
